vi "Check if Time to Log.vi"(0 "Data Log Times IN":u32[](array[numeric]), 1 "Data Log Rate (ms)":u32, 2 "Pumps Present":bool[](array[boolean])=[FALSE, FALSE, FALSE, FALSE, FALSE, FALSE], 3 "AKLH Log Times IN":u32[][](array[numeric]), 4 "AKLH Rate (ms)":u32, 5 "In Spec":bool[](array[boolean])=[FALSE, FALSE, FALSE, FALSE, FALSE, FALSE], 6 "Profile":string[][](array[string]), 7 "Current Step":i32=2, 8 "Pump Data":T1={"Voltages"=[0.015201568603515625, 0.00335693359375, 0.003021240234375, 0.12260055541992188, 0.06085968017578125, 0.052234649658203125], "PumpCurrent"=[0.015201568603515625, 0.00335693359375, 0.003021240234375, 0.12260055541992188, 0.06085968017578125, 0.052234649658203125], "Speed"=[0.0, 0.0, 0.0, 0.0, 0.0, 0.0], "ControllerCurrent"=[0.015201568603515625, 0.00335693359375, 0.003021240234375, 0.12260055541992188, 0.06085968017578125, 0.052234649658203125], "Pressure"=[0.015201568603515625, 0.00335693359375, 0.003021240234375, 0.12260055541992188, 0.06085968017578125, 0.052234649658203125], "Flow"=[0.0, 0.0, 0.0, 0.125, 0.0625, 0.0625], "Elapsed Time (Display)"=[7.1, 7.1, 7.1, 458133.45, 458138.85000000003, 458126.75], "Avg Pressure"=0.0, "Avg Speed"=0.0, "Elapsed Time"=[4074.9003000000002, 4074.9003000000002, 4074.9003000000002, 4074.9003000000002, 4074.9003000000002, 4074.9003000000002]} {"Elapsed Time" format="%<%H:%M:%S>t"; "Elapsed Time (Display)" format="%<%H:%M:%S>t"; "Speed" format="%#_4f"; "ControllerCurrent" format="%#.1g"; "Pressure" format="%#.0f"; "Flow" format="%#.0f"; "PumpCurrent" format="%#.1g"; "Voltages" format="%#.0f"}, 9 "Step Time Left":dbl=0.21101045608520508, 11 "Target Speeds":string[](array[string]), 13 "AKLH Filenames":string[](array[string])) -> (20 "Log Data":bool[](array[boolean]), 21 "Data Log Times OUT":u32[](array[numeric]), 22 "Log AKLH":bool[](array[boolean]), 23 "AKLH Log Times OUT":u32[][](array[numeric]), 24 "AKLH Filename":string, 25 "Target Speed":string)   [LabVIEW 2019]
uses:
  Controls/Pump Data.ctl
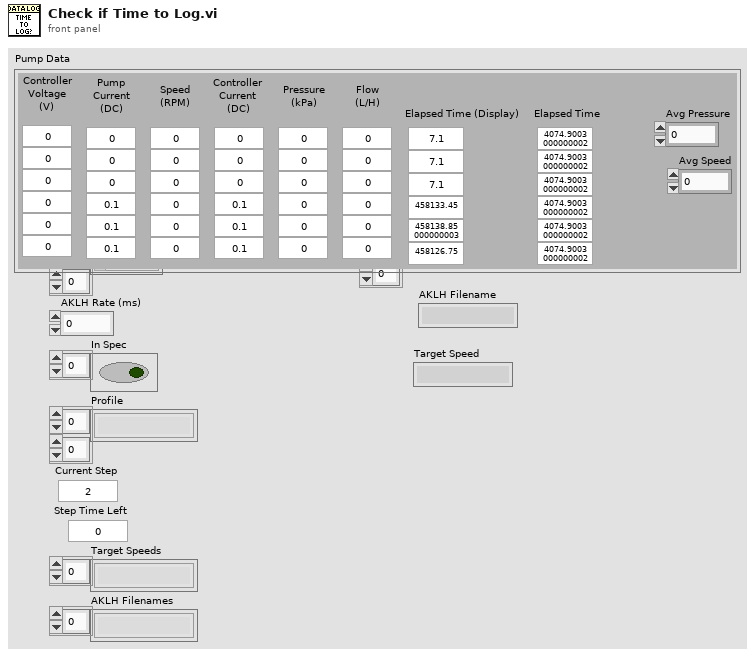
[diagram p1: front panel]
types:
  T1 = typedef "Pump Data.ctl" = cluster{"Voltages":dbl[], "PumpCurrent":dbl[], "Speed":dbl[], "ControllerCurrent":dbl[], "Pressure":dbl[], "Flow":dbl[], "Elapsed Time (Display)":dbl[], "Avg Pressure":dbl, "Avg Speed":dbl, "Elapsed Time":dbl[]}
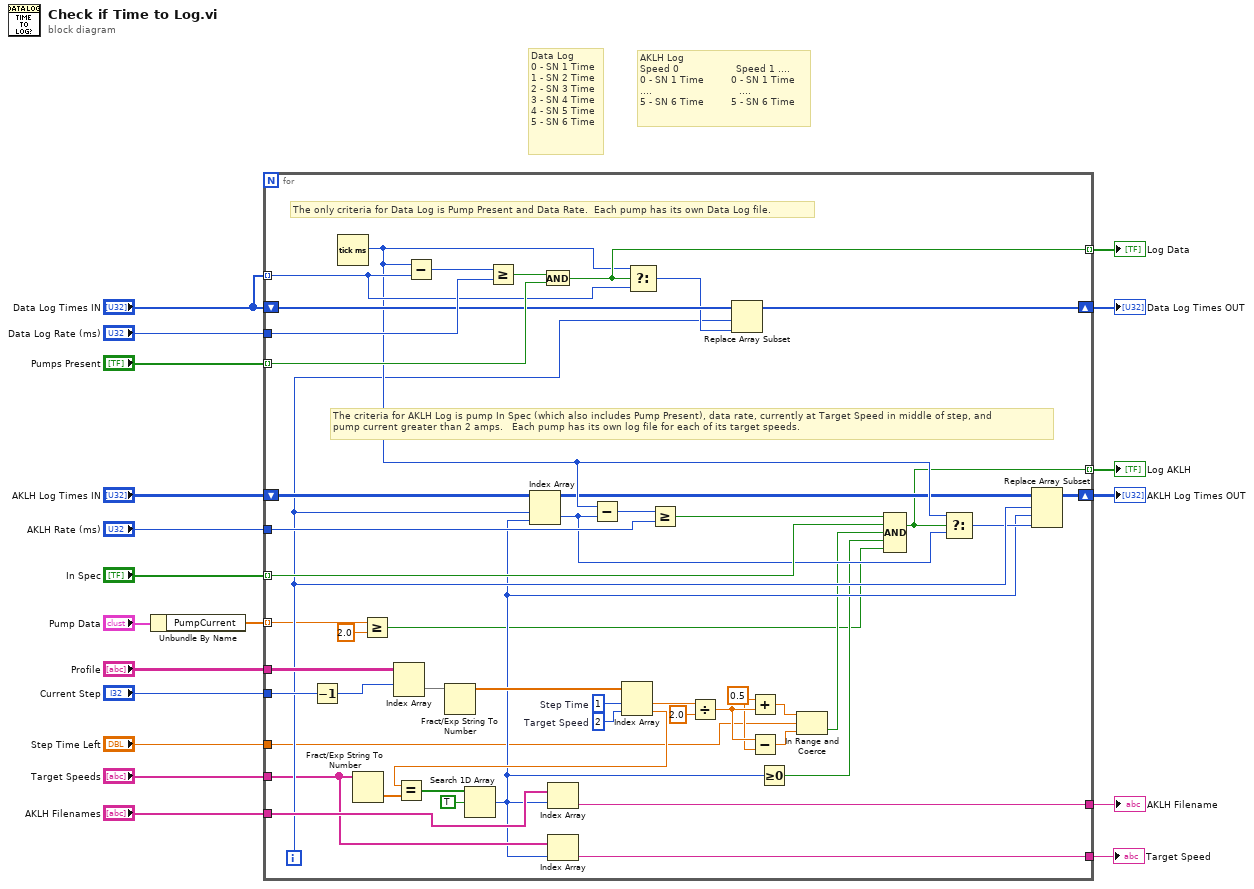
[diagram p0: block diagram]
diagram:
  # "AKLH Log\nSpeed 0                   Speed 1 ....\n0 - SN 1 Time         0 - SN 1 Time\n....                             ....\n5 - SN 6 Time         5 - SN 6 Time"
  # "Data Log\n0 - SN 1 Time\n1 - SN 2 Time\n2 - SN 3 Time\n3 - SN 4 Time\n4 - SN 5 Time\n5 - SN 6 Time"
  n1 = Unbundle By Name("Pump Data") -> ("PumpCurrent"=w1:dbl[])
  n2 = for {
    shift-right: [w60] -> w12
    shift-left: "Data Log Times IN" -> [w62]
    shift-right: [w36] -> w6
    shift-left: "AKLH Log Times IN" -> [w37]
    tunnel: "In Spec" -> [w40] mode=indexing
    tunnel: "Profile" -> [w58]
    tunnel: "Current Step" -> [w57]
    tunnel: "Step Time Left" -> [w24]
    tunnel: "Pumps Present" -> [w64] mode=indexing
    tunnel: "Data Log Times IN" -> [w63] mode=indexing
    tunnel: "Data Log Rate (ms)" -> [w66]
    tunnel: [w59] -> w11 mode=indexing
    tunnel: "Target Speeds" -> [w32]
    tunnel: "AKLH Filenames" -> [w45]
    tunnel: [w44] -> w8
    tunnel: "AKLH Rate (ms)" -> [w42]
    tunnel: [w33] -> w7 mode=indexing
    tunnel: [w31] -> w5
    tunnel: w1 -> [w22] mode=indexing
    i -> [w35]
    w27 = 0.5 ("y")
    w53 = 2  # Target Speed
    w55 = 1  # Step Time
    # "The criteria for AKLH Log is pump In Spec (which also includes Pump Present), data rate, currently at Target Speed in middle of step, and\npump current greater than 2 amps.   Each pump has its own log file for each of its target speeds."
    # "The only criteria for Data Log is Pump Present and Data Rate.  Each pump has its own Data Log file."
    n3 = Decrement(x=w57) -> (x-1=w54:i32)
    n4 = Tick Count (ms)() -> (millisecond timer value=w39:u32)
    n5 = Fract/Exp String To Number(string=w32) -> (number=w48:dbl[])  [unwired: 3 in, 1 out]
    n6 = Greater Or Equal?(x=w22, y=2.0) -> (x >= y?=w20:bool)
    n7 = Index Array(array=w58, index (row)=w54) -> (element=w56:string[])  [unwired: 1 in]
    n8 = Subtract(x=w39, y=w63) -> (x-y=w67:u32)
    n9 = Fract/Exp String To Number(string=w56) -> (number=w52:dbl[])  [unwired: 3 in, 1 out]
    n10 = Greater Or Equal?(x=w67, y=w66) -> (x >= y?=w65:bool)
    n11 = And(x=w65, y=w64) -> (x .and. y?=w59:bool)
    n12 = Index Array(array=w52, index #1=w55, index #2=w53) -> (element #1=w51:dbl, element #2=w49:dbl)
    n13 = Equal?(x=w49, y=w48) -> (x = y?=w47:bool[])
    n14 = Search 1D Array(1D array=w47, element=TRUE) -> (index of element=w30:i32)  [unwired: 1 in]
    n15 = Index Array(array=w37, index (row)=w35, index (col)=w30) -> (element=w38:u32)
    n16 = Index Array(array=w45, index=w30) -> (element=w44:string)
    n17 = Index Array(array=w32, index=w30) -> (element=w31:string)
    n18 = Subtract(x=w39, y=w38) -> (x-y=w43:u32)
    n19 = Select(t=w39, s=w59, f=w63) -> (s? t:f=w61:u32)
    n20 = Greater Or Equal?(x=w43, y=w42) -> (x >= y?=w41:bool)
    n21 = Divide(x=w51, y=2.0) -> (x/y=w28:dbl)
    n22 = Replace Array Subset(array=w62, new element=w61, index=w35) -> (w60:u32[])
    n23 = Add(x=w27, y=w28) -> (x+y=w26:dbl)
    n24 = Subtract(x=w28, y=w27) -> (x-y=w25:dbl)
    n25 = Greater Or Equal To 0?(x=w30) -> (x >= 0?=w29:bool)
    n26 = In Range and Coerce(upper limit=w26, x=w24, lower limit=w25) -> (In Range?=w23:bool)  [unwired: 1 out]
    n27 = Compound Arithmetic op=AND(w41, w40, w23, w29, w20) -> (w33:bool)
    n28 = Select(t=w39, s=w33, f=w38) -> (s? t:f=w34:u32)
    n29 = Replace Array Subset(array=w37, new element=w34, index (row)=w35, index (col)=w30) -> (w36:u32[][])
  }
  "Data Log Times OUT" <- w12
  "Log Data" <- w11
  "AKLH Filename" <- w8
  "Log AKLH" <- w7
  "AKLH Log Times OUT" <- w6
  "Target Speed" <- w5
